vi "Create Special Matrix.vi"   [LabVIEW 2020, in "NI_AALPro.lvlib"]
doc: "Generates a special matrix based on <B>matrix type</B>. The data types you wire to the <B>Input Vector2</B> and <B>Input Vector1</B> inputs determine the polymorphic instance to use."
uses:
  NI_AALPro.lvlib
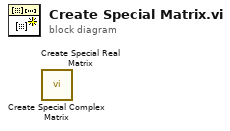
[diagram p0: block diagram]
diagram:
  n1 = call "Create Special Complex Matrix.vi"() -> ()  [unwired: 5 in, 2 out]
  n2 = call "Create Special Real Matrix.vi"() -> ()  [unwired: 5 in, 2 out]
